vi "Kbd_Event_key_demo(input).vi"() -> ()   [LabVIEW 2012]
panel:
  in  "string":string="1234AbCddFFfH"
  out "error out":errorcluster
  in  "error in":errorcluster
  in  "String":string
  # "1234AbCddFFfH"
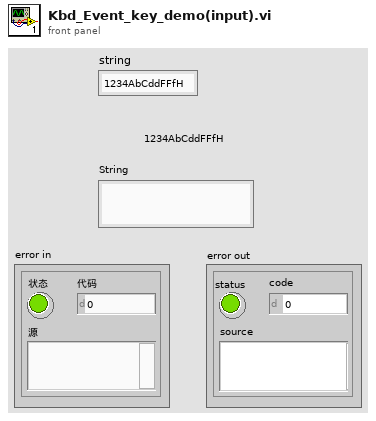
[diagram p1: front panel]
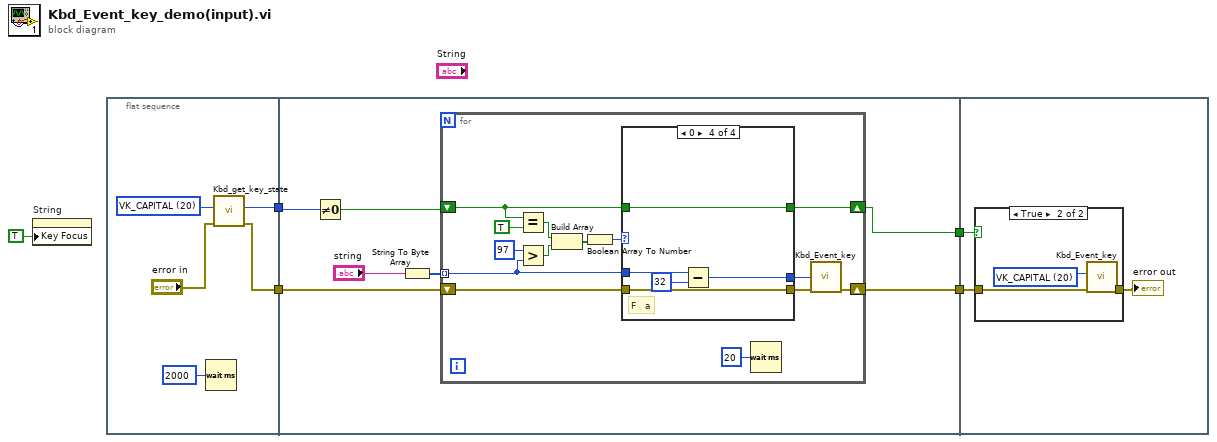
[diagram p0: block diagram]
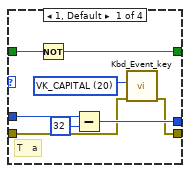
[diagram p2: hidden frame]
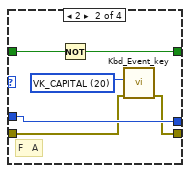
[diagram p3: hidden frame]
diagram:
  n1 = property on="String" class="Str"("Key Focus"=TRUE) -> ()  [unwired: 2 in, 2 out]
  n2 = flat-sequence {
    tunnel: [w8] -> w5
    tunnel: [w6] -> w2
    tunnel: w5 -> [w15]
    tunnel: [w13] -> w4
    tunnel: [w12] -> w3
    tunnel: w2 -> [w11]
    tunnel: w4 -> [w56]
    tunnel: w3 -> [w54]
    frame #0 {
      w9 = u8 20 items=["Undefined", "VK_LBUTTON", "VK_RBUTTON", "VK_CANCEL", "VK_MBUTTON", "VK_XBUTTON1", "VK_XBUTTON2", "Undefined", "VK_BACK", "VK_TAB", "Reserved", "Reserved", "VK_CLEAR", "VK_RETURN", "Undefined", "Undefined", "VK_SHIFT", "VK_CONTROL", "VK_MENU", "VK_PAUSE", "VK_CAPITAL", "VK_KANA", "Undefined", "VK_JUNJA", "VK_FINAL", "VK_HANJA", "Undefined", "VK_ESCAPE", "VK_CONVERT", "VK_NONCONVERT", "VK_ACCEPT", "VK_MODECHANGE", "VK_SPACE", "VK_PRIOR", "VK_NEXT", "VK_END", "VK_HOME", "VK_LEFT", "VK_UP", "VK_RIGHT", "VK_DOWN", "VK_SELECT", "VK_PRINT", "VK_EXECUTE", "VK_SNAPSHOT", "VK_INSERT", "VK_DELETE", "VK_HELP", "VK_0", "VK_1", "VK_2", "VK_3", "VK_4", "VK_5", "VK_6", "VK_7", "VK_8", "VK_9", "Undefined", "Undefined", "Undefined", "Undefined", "Undefined", "Undefined", "Undefined", "VK_A", "VK_B", "VK_C", "VK_D", "VK_E", "VK_F", "VK_G", "VK_H", "VK_I", "VK_J", "VK_K", "VK_L", "VK_M", "VK_N", "VK_O", "VK_P", "VK_Q", "VK_R", "VK_S", "VK_T", "VK_U", "VK_V", "VK_W", "VK_X", "VK_Y", "VK_Z", "VK_LWIN", "VK_RWIN", "VK_APPS", "Reserved", "VK_SLEEP", "VK_NUMPAD0", "VK_NUMPAD1", "VK_NUMPAD2", "VK_NUMPAD3", "VK_NUMPAD4", "VK_NUMPAD5", "VK_NUMPAD6", "VK_NUMPAD7", "VK_NUMPAD8", "VK_NUMPAD9", "VK_MULTIPLY", "VK_ADD", "VK_SEPARATOR", "VK_SUBTRACT", "VK_DECIMAL", "VK_DIVIDE", "VK_F1", "VK_F2", "VK_F3", "VK_F4", "VK_F5", "VK_F6", "VK_F7", "VK_F8", "VK_F9", "VK_F10", "VK_F11", "VK_F12", "VK_F13", "VK_F14", "VK_F15", "VK_F16", "VK_F17", "VK_F18", "VK_F19  ", "VK_F20 ", "VK_F21", "VK_F22 ", "VK_F23", "VK_F24", "Unsigned", "Unsigned", "Unsigned", "Unsigned", "Unsigned", "Unsigned", "Unsigned", "Unsigned", "VK_NUMLOCK", "VK_SCROLL", "OEM Specific", " OEM Speicfic", "OEM Speicfic", "OEM Specific", "OEM Specific", "Unassigned", "Unassigned", "Unassigned", "Unassigned", "Unassigned", "Unassigned", "Unassigned", "Unassigned", "Unassigned", "VK_LSHIFT", "VK_RSHIFT", "VK_LCONTROL", "VK_RCONTROL", "VK_LMENU", "VK_RMENU", "VK_BROWSER_BACK", "VK_BROWSER_FORWARD", "VK_BROWSER_REFRESH", "VK_BROWSER_STOP", "VK_BROWSER_SEARCH", "VK_BROWSER_FAVORITES ", "VK_BROWSER_HOME", "VK_VOLUME_MUTE", "VK_VOLUME_DOWN", "VK_VOLUME_UP", "VK_MEDIA_NEXT_TRACK", "VK_MEDIA_PREV_TRACK", "VK_MEDIA_STOP ", "VK_MEDIA_PLAY_PAUSE", "VK_LAUNCH_MAIL", "VK_LAUNCH_MEDIA_SELECT", "VK_LAUNCH_APP1", "VK_LAUNCH_APP2", "Reserved", "Reserved", "VK_OEM_1(;:)", "VK_OEM_PLUS(+) ", "VK_OEM_COMMA(,)", "VK_OEM_MINUS(-)", "VK_OEM_PERIOD(.)", "VK_OEM_2(/?)", "VK_OEM_3(~`)", "Reserved", "Reserved", "Reserved", "Reserved", "Reserved", "Reserved", "Reserved", "Reserved", "Reserved", "Reserved", "Reserved", "Reserved", "Reserved", "Reserved", "Reserved", "Reserved", "Reserved", "Reserved", "Reserved", "Reserved", "Reserved", "Reserved", "Reserved", "Reserved", "Reserved", "Reserved", "VK_OEM_4 ([{)", "VK_OEM_5 (\\|)", "VK_OEM_6 (]})", "VK_OEM_7 ('\")", "VK_OEM_8", "Reserved", "Reserved", "VK_OEM_102", "OEM Specific", "OEM Specific", "VK_PROCESSKEY", "OEM Specific", "VK_PACKET", "Unassigned", "OEM Specific", "OEM Specific", "OEM Specific", "OEM Specific", "OEM Specific", "OEM Specific", "OEM Specific", "OEM Specific", "OEM Specific", "OEM Specific", "OEM Specific", "OEM Specific", "OEM Specific", "VK_ATTN", "VK_CRSEL", "VK_EXSEL", "VK_EREOF", "VK_PLAY", "VK_ZOOM", "VK_NONAME", "VK_PA1", "VK_OEM_CLEAR "] ("VK_CODE")
      n3 = Wait (ms)(milliseconds to wait=u32 2000) -> ()  [unwired: 1 out]
      n4 = call "Kbd_get_key_state.vi"("error in"="error in", "VK_CODE"=w9) -> ("error out"=w6:errorcluster, "return type"=w8:u8)  [unwired: 8 in]
    }
    frame #1 {
      n5 = Not Equal To 0?(x=w15) -> (x != 0?=w14:bool)
      n6 = String To Byte Array(string="string") -> (unsigned byte array=w17:u8[])
      n7 = for {
        tunnel: w17 -> [w26] mode=indexing
        shift-right: [w31] -> w13
        shift-left: w11 -> [w19]
        shift-right: [w28] -> w12
        shift-left: w14 -> [w27]
        n8 = Equal?(x=w27, y=TRUE) -> (x = y?=w24:bool)
        n9 = Greater?(x=u8 97, y=w26) -> (0:w20:bool)
        n10 = Build Array(w24, w20) -> (w23:bool[])
        n11 = Boolean Array To Number(Boolean array=w23) -> (number=w22:u32)
        n12 = case shown="0" w22 {
          tunnel: w27 -> [w38 w44 w48 w53]
          tunnel: [w37 w43 w48 w53] -> w28
          tunnel: w26 -> [w36 w42 w47 w52]
          tunnel: [w34 w42 w47 w50] -> w25
          tunnel: w19 -> [w33 w41 w46 w49]
          tunnel: [w32 w40 w46 w49] -> w18
          frame 1, Default {
            w39 = u8 20 items=["Undefined", "VK_LBUTTON", "VK_RBUTTON", "VK_CANCEL", "VK_MBUTTON", "VK_XBUTTON1", "VK_XBUTTON2", "Undefined", "VK_BACK", "VK_TAB", "Reserved", "Reserved", "VK_CLEAR", "VK_RETURN", "Undefined", "Undefined", "VK_SHIFT", "VK_CONTROL", "VK_MENU", "VK_PAUSE", "VK_CAPITAL", "VK_KANA", "Undefined", "VK_JUNJA", "VK_FINAL", "VK_HANJA", "Undefined", "VK_ESCAPE", "VK_CONVERT", "VK_NONCONVERT", "VK_ACCEPT", "VK_MODECHANGE", "VK_SPACE", "VK_PRIOR", "VK_NEXT", "VK_END", "VK_HOME", "VK_LEFT", "VK_UP", "VK_RIGHT", "VK_DOWN", "VK_SELECT", "VK_PRINT", "VK_EXECUTE", "VK_SNAPSHOT", "VK_INSERT", "VK_DELETE", "VK_HELP", "VK_0", "VK_1", "VK_2", "VK_3", "VK_4", "VK_5", "VK_6", "VK_7", "VK_8", "VK_9", "Undefined", "Undefined", "Undefined", "Undefined", "Undefined", "Undefined", "Undefined", "VK_A", "VK_B", "VK_C", "VK_D", "VK_E", "VK_F", "VK_G", "VK_H", "VK_I", "VK_J", "VK_K", "VK_L", "VK_M", "VK_N", "VK_O", "VK_P", "VK_Q", "VK_R", "VK_S", "VK_T", "VK_U", "VK_V", "VK_W", "VK_X", "VK_Y", "VK_Z", "VK_LWIN", "VK_RWIN", "VK_APPS", "Reserved", "VK_SLEEP", "VK_NUMPAD0", "VK_NUMPAD1", "VK_NUMPAD2", "VK_NUMPAD3", "VK_NUMPAD4", "VK_NUMPAD5", "VK_NUMPAD6", "VK_NUMPAD7", "VK_NUMPAD8", "VK_NUMPAD9", "VK_MULTIPLY", "VK_ADD", "VK_SEPARATOR", "VK_SUBTRACT", "VK_DECIMAL", "VK_DIVIDE", "VK_F1", "VK_F2", "VK_F3", "VK_F4", "VK_F5", "VK_F6", "VK_F7", "VK_F8", "VK_F9", "VK_F10", "VK_F11", "VK_F12", "VK_F13", "VK_F14", "VK_F15", "VK_F16", "VK_F17", "VK_F18", "VK_F19  ", "VK_F20 ", "VK_F21", "VK_F22 ", "VK_F23", "VK_F24", "Unsigned", "Unsigned", "Unsigned", "Unsigned", "Unsigned", "Unsigned", "Unsigned", "Unsigned", "VK_NUMLOCK", "VK_SCROLL", "OEM Specific", " OEM Speicfic", "OEM Speicfic", "OEM Specific", "OEM Specific", "Unassigned", "Unassigned", "Unassigned", "Unassigned", "Unassigned", "Unassigned", "Unassigned", "Unassigned", "Unassigned", "VK_LSHIFT", "VK_RSHIFT", "VK_LCONTROL", "VK_RCONTROL", "VK_LMENU", "VK_RMENU", "VK_BROWSER_BACK", "VK_BROWSER_FORWARD", "VK_BROWSER_REFRESH", "VK_BROWSER_STOP", "VK_BROWSER_SEARCH", "VK_BROWSER_FAVORITES ", "VK_BROWSER_HOME", "VK_VOLUME_MUTE", "VK_VOLUME_DOWN", "VK_VOLUME_UP", "VK_MEDIA_NEXT_TRACK", "VK_MEDIA_PREV_TRACK", "VK_MEDIA_STOP ", "VK_MEDIA_PLAY_PAUSE", "VK_LAUNCH_MAIL", "VK_LAUNCH_MEDIA_SELECT", "VK_LAUNCH_APP1", "VK_LAUNCH_APP2", "Reserved", "Reserved", "VK_OEM_1(;:)", "VK_OEM_PLUS(+) ", "VK_OEM_COMMA(,)", "VK_OEM_MINUS(-)", "VK_OEM_PERIOD(.)", "VK_OEM_2(/?)", "VK_OEM_3(~`)", "Reserved", "Reserved", "Reserved", "Reserved", "Reserved", "Reserved", "Reserved", "Reserved", "Reserved", "Reserved", "Reserved", "Reserved", "Reserved", "Reserved", "Reserved", "Reserved", "Reserved", "Reserved", "Reserved", "Reserved", "Reserved", "Reserved", "Reserved", "Reserved", "Reserved", "Reserved", "VK_OEM_4 ([{)", "VK_OEM_5 (\\|)", "VK_OEM_6 (]})", "VK_OEM_7 ('\")", "VK_OEM_8", "Reserved", "Reserved", "VK_OEM_102", "OEM Specific", "OEM Specific", "VK_PROCESSKEY", "OEM Specific", "VK_PACKET", "Unassigned", "OEM Specific", "OEM Specific", "OEM Specific", "OEM Specific", "OEM Specific", "OEM Specific", "OEM Specific", "OEM Specific", "OEM Specific", "OEM Specific", "OEM Specific", "OEM Specific", "OEM Specific", "VK_ATTN", "VK_CRSEL", "VK_EXSEL", "VK_EREOF", "VK_PLAY", "VK_ZOOM", "VK_NONAME", "VK_PA1", "VK_OEM_CLEAR "] ("VK_CODE")
            # "T   a"
            n13 = Not(x=w38) -> (.not. x?=w37:bool)
            n14 = Subtract(x=w36, y=u8 32) -> (x-y=w34:u8)
            n15 = call "Kbd_Event_key.vi"("error in"=w33, "VK_CODE"=w39) -> ("error out"=w32:errorcluster)  [unwired: 9 in]
          }
          frame 2 {
            w45 = u8 20 items=["Undefined", "VK_LBUTTON", "VK_RBUTTON", "VK_CANCEL", "VK_MBUTTON", "VK_XBUTTON1", "VK_XBUTTON2", "Undefined", "VK_BACK", "VK_TAB", "Reserved", "Reserved", "VK_CLEAR", "VK_RETURN", "Undefined", "Undefined", "VK_SHIFT", "VK_CONTROL", "VK_MENU", "VK_PAUSE", "VK_CAPITAL", "VK_KANA", "Undefined", "VK_JUNJA", "VK_FINAL", "VK_HANJA", "Undefined", "VK_ESCAPE", "VK_CONVERT", "VK_NONCONVERT", "VK_ACCEPT", "VK_MODECHANGE", "VK_SPACE", "VK_PRIOR", "VK_NEXT", "VK_END", "VK_HOME", "VK_LEFT", "VK_UP", "VK_RIGHT", "VK_DOWN", "VK_SELECT", "VK_PRINT", "VK_EXECUTE", "VK_SNAPSHOT", "VK_INSERT", "VK_DELETE", "VK_HELP", "VK_0", "VK_1", "VK_2", "VK_3", "VK_4", "VK_5", "VK_6", "VK_7", "VK_8", "VK_9", "Undefined", "Undefined", "Undefined", "Undefined", "Undefined", "Undefined", "Undefined", "VK_A", "VK_B", "VK_C", "VK_D", "VK_E", "VK_F", "VK_G", "VK_H", "VK_I", "VK_J", "VK_K", "VK_L", "VK_M", "VK_N", "VK_O", "VK_P", "VK_Q", "VK_R", "VK_S", "VK_T", "VK_U", "VK_V", "VK_W", "VK_X", "VK_Y", "VK_Z", "VK_LWIN", "VK_RWIN", "VK_APPS", "Reserved", "VK_SLEEP", "VK_NUMPAD0", "VK_NUMPAD1", "VK_NUMPAD2", "VK_NUMPAD3", "VK_NUMPAD4", "VK_NUMPAD5", "VK_NUMPAD6", "VK_NUMPAD7", "VK_NUMPAD8", "VK_NUMPAD9", "VK_MULTIPLY", "VK_ADD", "VK_SEPARATOR", "VK_SUBTRACT", "VK_DECIMAL", "VK_DIVIDE", "VK_F1", "VK_F2", "VK_F3", "VK_F4", "VK_F5", "VK_F6", "VK_F7", "VK_F8", "VK_F9", "VK_F10", "VK_F11", "VK_F12", "VK_F13", "VK_F14", "VK_F15", "VK_F16", "VK_F17", "VK_F18", "VK_F19  ", "VK_F20 ", "VK_F21", "VK_F22 ", "VK_F23", "VK_F24", "Unsigned", "Unsigned", "Unsigned", "Unsigned", "Unsigned", "Unsigned", "Unsigned", "Unsigned", "VK_NUMLOCK", "VK_SCROLL", "OEM Specific", " OEM Speicfic", "OEM Speicfic", "OEM Specific", "OEM Specific", "Unassigned", "Unassigned", "Unassigned", "Unassigned", "Unassigned", "Unassigned", "Unassigned", "Unassigned", "Unassigned", "VK_LSHIFT", "VK_RSHIFT", "VK_LCONTROL", "VK_RCONTROL", "VK_LMENU", "VK_RMENU", "VK_BROWSER_BACK", "VK_BROWSER_FORWARD", "VK_BROWSER_REFRESH", "VK_BROWSER_STOP", "VK_BROWSER_SEARCH", "VK_BROWSER_FAVORITES ", "VK_BROWSER_HOME", "VK_VOLUME_MUTE", "VK_VOLUME_DOWN", "VK_VOLUME_UP", "VK_MEDIA_NEXT_TRACK", "VK_MEDIA_PREV_TRACK", "VK_MEDIA_STOP ", "VK_MEDIA_PLAY_PAUSE", "VK_LAUNCH_MAIL", "VK_LAUNCH_MEDIA_SELECT", "VK_LAUNCH_APP1", "VK_LAUNCH_APP2", "Reserved", "Reserved", "VK_OEM_1(;:)", "VK_OEM_PLUS(+) ", "VK_OEM_COMMA(,)", "VK_OEM_MINUS(-)", "VK_OEM_PERIOD(.)", "VK_OEM_2(/?)", "VK_OEM_3(~`)", "Reserved", "Reserved", "Reserved", "Reserved", "Reserved", "Reserved", "Reserved", "Reserved", "Reserved", "Reserved", "Reserved", "Reserved", "Reserved", "Reserved", "Reserved", "Reserved", "Reserved", "Reserved", "Reserved", "Reserved", "Reserved", "Reserved", "Reserved", "Reserved", "Reserved", "Reserved", "VK_OEM_4 ([{)", "VK_OEM_5 (\\|)", "VK_OEM_6 (]})", "VK_OEM_7 ('\")", "VK_OEM_8", "Reserved", "Reserved", "VK_OEM_102", "OEM Specific", "OEM Specific", "VK_PROCESSKEY", "OEM Specific", "VK_PACKET", "Unassigned", "OEM Specific", "OEM Specific", "OEM Specific", "OEM Specific", "OEM Specific", "OEM Specific", "OEM Specific", "OEM Specific", "OEM Specific", "OEM Specific", "OEM Specific", "OEM Specific", "OEM Specific", "VK_ATTN", "VK_CRSEL", "VK_EXSEL", "VK_EREOF", "VK_PLAY", "VK_ZOOM", "VK_NONAME", "VK_PA1", "VK_OEM_CLEAR "] ("VK_CODE")
            # "F   A"
            n16 = Not(x=w44) -> (.not. x?=w43:bool)
            n17 = call "Kbd_Event_key.vi"("error in"=w41, "VK_CODE"=w45) -> ("error out"=w40:errorcluster)  [unwired: 9 in]
          }
          frame 3 {
            # "T   A"
          }
          frame 0 {
            # "F   a"
            n18 = Subtract(x=w52, y=u8 32) -> (x-y=w50:u8)
          }
        }
        n19 = Wait (ms)(milliseconds to wait=u32 20) -> ()  [unwired: 1 out]
        n20 = call "Kbd_Event_key.vi"("error in"=w18, "VK_CODE"=w25) -> ("error out"=w31:errorcluster)  [unwired: 9 in]
      }
    }
    frame #2 {
      n21 = case shown="True" w54 {
        tunnel: w56 -> [w57 w59]
        tunnel: [w57 w58] -> w55
        frame False {
        }
        frame True {
          w60 = u8 20 items=["Undefined", "VK_LBUTTON", "VK_RBUTTON", "VK_CANCEL", "VK_MBUTTON", "VK_XBUTTON1", "VK_XBUTTON2", "Undefined", "VK_BACK", "VK_TAB", "Reserved", "Reserved", "VK_CLEAR", "VK_RETURN", "Undefined", "Undefined", "VK_SHIFT", "VK_CONTROL", "VK_MENU", "VK_PAUSE", "VK_CAPITAL", "VK_KANA", "Undefined", "VK_JUNJA", "VK_FINAL", "VK_HANJA", "Undefined", "VK_ESCAPE", "VK_CONVERT", "VK_NONCONVERT", "VK_ACCEPT", "VK_MODECHANGE", "VK_SPACE", "VK_PRIOR", "VK_NEXT", "VK_END", "VK_HOME", "VK_LEFT", "VK_UP", "VK_RIGHT", "VK_DOWN", "VK_SELECT", "VK_PRINT", "VK_EXECUTE", "VK_SNAPSHOT", "VK_INSERT", "VK_DELETE", "VK_HELP", "VK_0", "VK_1", "VK_2", "VK_3", "VK_4", "VK_5", "VK_6", "VK_7", "VK_8", "VK_9", "Undefined", "Undefined", "Undefined", "Undefined", "Undefined", "Undefined", "Undefined", "VK_A", "VK_B", "VK_C", "VK_D", "VK_E", "VK_F", "VK_G", "VK_H", "VK_I", "VK_J", "VK_K", "VK_L", "VK_M", "VK_N", "VK_O", "VK_P", "VK_Q", "VK_R", "VK_S", "VK_T", "VK_U", "VK_V", "VK_W", "VK_X", "VK_Y", "VK_Z", "VK_LWIN", "VK_RWIN", "VK_APPS", "Reserved", "VK_SLEEP", "VK_NUMPAD0", "VK_NUMPAD1", "VK_NUMPAD2", "VK_NUMPAD3", "VK_NUMPAD4", "VK_NUMPAD5", "VK_NUMPAD6", "VK_NUMPAD7", "VK_NUMPAD8", "VK_NUMPAD9", "VK_MULTIPLY", "VK_ADD", "VK_SEPARATOR", "VK_SUBTRACT", "VK_DECIMAL", "VK_DIVIDE", "VK_F1", "VK_F2", "VK_F3", "VK_F4", "VK_F5", "VK_F6", "VK_F7", "VK_F8", "VK_F9", "VK_F10", "VK_F11", "VK_F12", "VK_F13", "VK_F14", "VK_F15", "VK_F16", "VK_F17", "VK_F18", "VK_F19  ", "VK_F20 ", "VK_F21", "VK_F22 ", "VK_F23", "VK_F24", "Unsigned", "Unsigned", "Unsigned", "Unsigned", "Unsigned", "Unsigned", "Unsigned", "Unsigned", "VK_NUMLOCK", "VK_SCROLL", "OEM Specific", " OEM Speicfic", "OEM Speicfic", "OEM Specific", "OEM Specific", "Unassigned", "Unassigned", "Unassigned", "Unassigned", "Unassigned", "Unassigned", "Unassigned", "Unassigned", "Unassigned", "VK_LSHIFT", "VK_RSHIFT", "VK_LCONTROL", "VK_RCONTROL", "VK_LMENU", "VK_RMENU", "VK_BROWSER_BACK", "VK_BROWSER_FORWARD", "VK_BROWSER_REFRESH", "VK_BROWSER_STOP", "VK_BROWSER_SEARCH", "VK_BROWSER_FAVORITES ", "VK_BROWSER_HOME", "VK_VOLUME_MUTE", "VK_VOLUME_DOWN", "VK_VOLUME_UP", "VK_MEDIA_NEXT_TRACK", "VK_MEDIA_PREV_TRACK", "VK_MEDIA_STOP ", "VK_MEDIA_PLAY_PAUSE", "VK_LAUNCH_MAIL", "VK_LAUNCH_MEDIA_SELECT", "VK_LAUNCH_APP1", "VK_LAUNCH_APP2", "Reserved", "Reserved", "VK_OEM_1(;:)", "VK_OEM_PLUS(+) ", "VK_OEM_COMMA(,)", "VK_OEM_MINUS(-)", "VK_OEM_PERIOD(.)", "VK_OEM_2(/?)", "VK_OEM_3(~`)", "Reserved", "Reserved", "Reserved", "Reserved", "Reserved", "Reserved", "Reserved", "Reserved", "Reserved", "Reserved", "Reserved", "Reserved", "Reserved", "Reserved", "Reserved", "Reserved", "Reserved", "Reserved", "Reserved", "Reserved", "Reserved", "Reserved", "Reserved", "Reserved", "Reserved", "Reserved", "VK_OEM_4 ([{)", "VK_OEM_5 (\\|)", "VK_OEM_6 (]})", "VK_OEM_7 ('\")", "VK_OEM_8", "Reserved", "Reserved", "VK_OEM_102", "OEM Specific", "OEM Specific", "VK_PROCESSKEY", "OEM Specific", "VK_PACKET", "Unassigned", "OEM Specific", "OEM Specific", "OEM Specific", "OEM Specific", "OEM Specific", "OEM Specific", "OEM Specific", "OEM Specific", "OEM Specific", "OEM Specific", "OEM Specific", "OEM Specific", "OEM Specific", "VK_ATTN", "VK_CRSEL", "VK_EXSEL", "VK_EREOF", "VK_PLAY", "VK_ZOOM", "VK_NONAME", "VK_PA1", "VK_OEM_CLEAR "] ("VK_CODE")
          n22 = call "Kbd_Event_key.vi"("error in"=w59, "VK_CODE"=w60) -> ("error out"=w58:errorcluster)  [unwired: 9 in]
        }
      }
      "error out" <- w55
    }
  }
